vi "Custom Assertion Failure Message.vi"() -> ()   [LabVIEW 2017, in "Transparent Assertions.Tests.lvlib" / "Assert Error Message Contains String.lvlib"]
uses:
  Assert Error Message Contains String.lvlib
  src/Transparent Assertions/Transparent Assertions.lvlib
  Transparent Assertions.Tests.lvlib
panel:
  out "error out":errorcluster
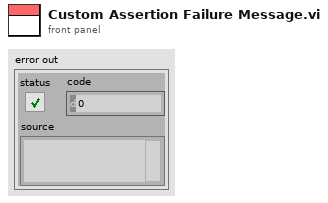
[diagram p1: front panel]
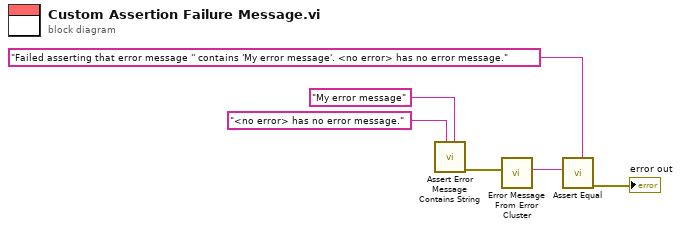
[diagram p0: block diagram]
diagram:
  n1 = call "Assert Error Message Contains String.vi"("Expected"="My error message", "Message (\"\")"="<no error> has no error message." ("Message (\"\")")) -> ("error out"=w2:errorcluster)  [unwired: 9 in]
  n2 = call "Error Message From Error Cluster.vi"("Error"=w2) -> ("Error Message"=w1:string)  [unwired: 10 in]
  n3 = call "Assert Equal.vi"("Expected"="Failed asserting that error message '' contains 'My error message'. <no error> has no error message." ("Needle"), "Actual"=w1) -> ("error out"=→"error out":errorcluster)  [unwired: 9 in]
